vi "CRYCalcu Arithmetic Value.vi"(4 "dB ref":dbl format="%#_6p", 5 "Axis Mode":u16(slide), 6 "B data for units":T1={"Name"="", "Curve"=[], "X data"=1, "Y data"=1, "Z data"=1, "X axis"=0, "Y axis"=1, "Z axis"=1, "X unit"="Hz", "Y unit"="", "Z unit"="deg.", "X dB ref"=1.0, "Y dB ref"=1.0, "Z dB ref"=1.0, "single val"=FALSE, "protected"=FALSE, "display X"=TRUE, "display Y"=TRUE, "display Z"=TRUE, "Test Info"="", "Step No."=0, "Plot Settings"={"Color"=0, "Interpolation"=0, "Point Style"=0, "Line Style"=0, "Point Color"=0, "Line Width"=0, "Bar Plot Style"=0, "Fill To"=0}, "AutoProtect"=FALSE} {"Z data" items=["dB", "Lin"]; "X data" items=["dB", "Lin"]; "Y data" items=["dB", "Lin"]; "Z dB ref" format="%.1f"; "Z axis" items=["Log", "Lin"]; "X dB ref" format="%.1f"; "X axis" items=["Log", "Lin"]; "Y axis" items=["Log", "Lin"]; "Y dB ref" format="%.1f"; "Curve"."z" format="%.2f"; "Curve"."y" format="%.2f"; "Curve"."x" format="%.2f"}, 7 "A data for units":T1={"Name"="", "Curve"=[], "X data"=1, "Y data"=1, "Z data"=1, "X axis"=0, "Y axis"=1, "Z axis"=1, "X unit"="Hz", "Y unit"="", "Z unit"="deg.", "X dB ref"=1.0, "Y dB ref"=1.0, "Z dB ref"=1.0, "single val"=FALSE, "protected"=FALSE, "display X"=TRUE, "display Y"=TRUE, "display Z"=TRUE, "Test Info"="", "Step No."=0, "Plot Settings"={"Color"=0, "Interpolation"=0, "Point Style"=0, "Line Style"=0, "Point Color"=0, "Line Width"=0, "Bar Plot Style"=0, "Fill To"=0}, "AutoProtect"=FALSE} {"Z data" items=["dB", "Lin"]; "X data" items=["dB", "Lin"]; "Y data" items=["dB", "Lin"]; "Z dB ref" format="%.1f"; "Z axis" items=["Log", "Lin"]; "X dB ref" format="%.1f"; "X axis" items=["Log", "Lin"]; "Y axis" items=["Log", "Lin"]; "Y dB ref" format="%.1f"; "Curve"."z" format="%.2f"; "Curve"."y" format="%.2f"; "Curve"."x" format="%.2f"}, 8 "Curve B":cluster{"x":dbl, "y":dbl, "z":dbl}[](array[cluster]) {"z" format="%.2f"; "y" format="%.2f"; "x" format="%.2f"}, 9 "operator":u16(ring) items=["+", "--", "x", "/"], 10 "Work in":u16(slide), 11 "Curve A":cluster{"x":dbl, "y":dbl, "z":dbl}[](array[cluster]) {"z" format="%.2f"; "y" format="%.2f"; "x" format="%.2f"}) -> (2 "Result":cluster{"x":dbl, "y":dbl, "z":dbl}[](array[cluster]) {"z" format="%.2f"; "y" format="%.2f"; "x" format="%.2f"})   [LabVIEW 2013]
uses:
  Typedef Control/CRYData Cluster.ctl
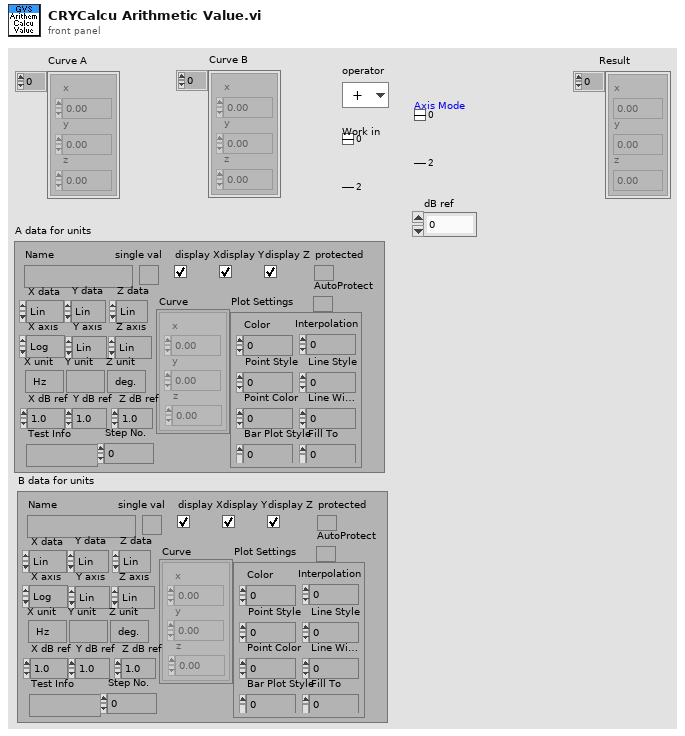
[diagram p1: front panel]
types:
  T1 = typedef "CRYData Cluster.ctl" = cluster{"Name":string, "Curve":cluster{"x":dbl, "y":dbl, "z":dbl}[], "X data":u16, "Y data":u16, "Z data":u16, "X axis":u16, "Y axis":u16, "Z axis":u16, "X unit":string, "Y unit":string, "Z unit":string, "X dB ref":dbl, "Y dB ref":dbl, "Z dB ref":dbl, "single val":bool, "protected":bool, "display X":bool, "display Y":bool, "display Z":bool, "Test Info":string, "Step No.":i32, "Plot Settings":cluster{"Color":u32, "Interpolation":u8, "Point Style":u8, "Line Style":u8, "Point Color":u32, "Line Width":u8, "Bar Plot Style":u8, "Fill To":i16}, "AutoProtect":bool}
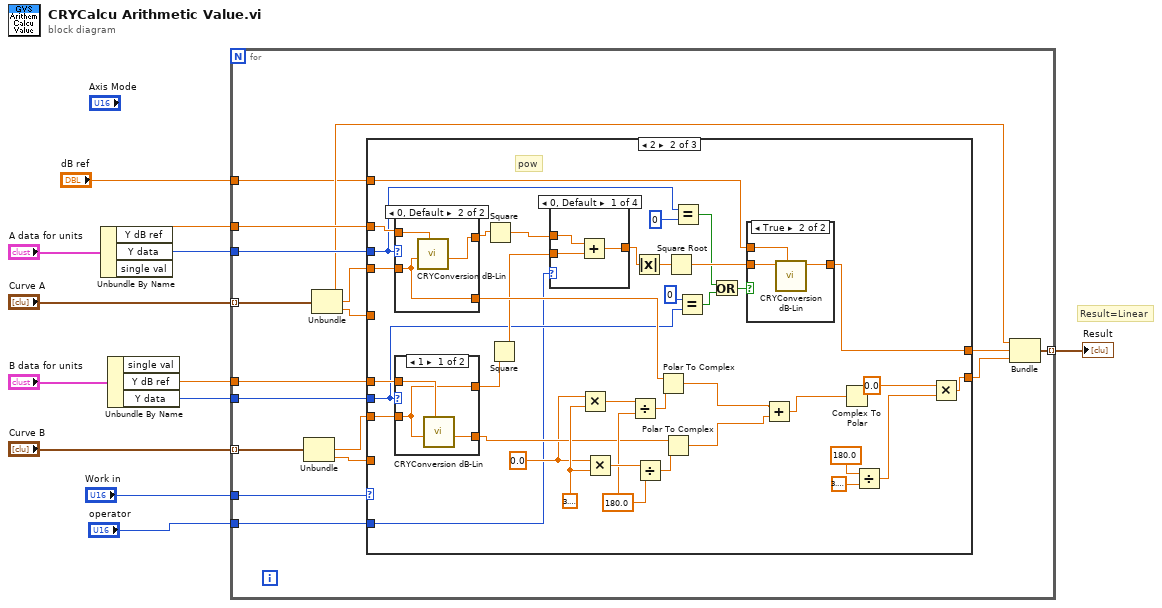
[diagram p0: block diagram]
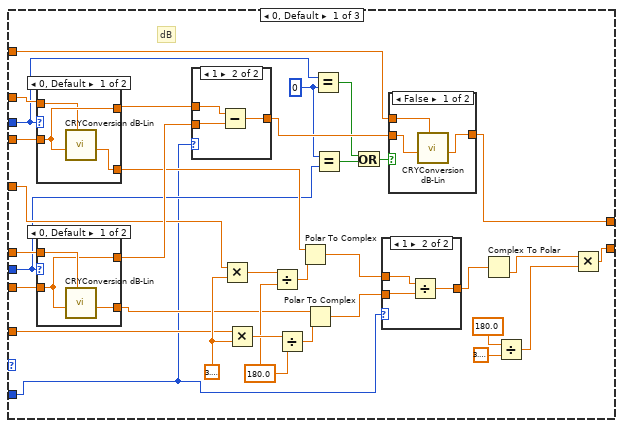
[diagram p2: hidden frame]
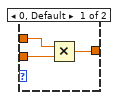
[diagram p4: hidden frame]
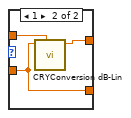
[diagram p5: hidden frame]
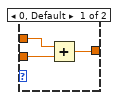
[diagram p6: hidden frame]
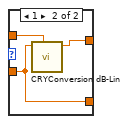
[diagram p7: hidden frame]
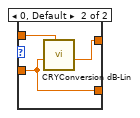
[diagram p9: hidden frame]
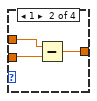
[diagram p10: hidden frame]
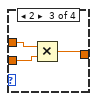
[diagram p11: hidden frame]
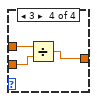
[diagram p12: hidden frame]
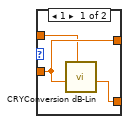
[diagram p13: hidden frame]
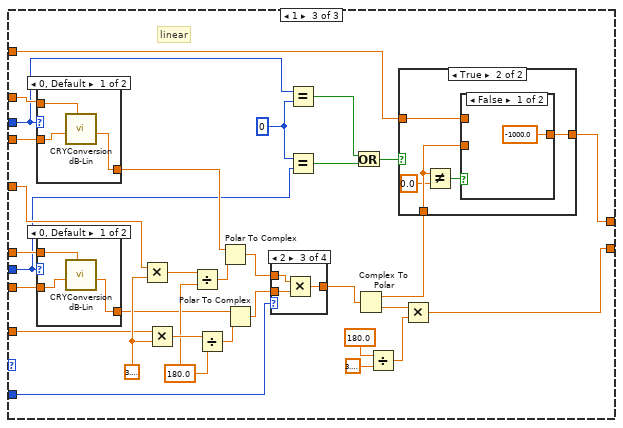
[diagram p14: hidden frame]
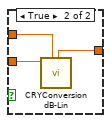
[diagram p16: hidden frame]
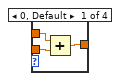
[diagram p17: hidden frame]
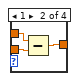
[diagram p18: hidden frame]
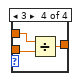
[diagram p19: hidden frame]
diagram:
  # "Result=Linear"
  n1 = Unbundle By Name("A data for units") -> ("Y dB ref"=w6:dbl, "Y data"=w7:u16)  [unwired: 1 out]
  n2 = Unbundle By Name("B data for units") -> ("Y dB ref"=w4:dbl, "Y data"=w5:u16)  [unwired: 1 out]
  n3 = for {
    tunnel: "Curve B" -> [w29] mode=indexing
    tunnel: "Curve A" -> [w28] mode=indexing
    tunnel: [w27] -> w11 mode=indexing
    tunnel: w7 -> [w26]
    tunnel: w6 -> [w25]
    tunnel: w5 -> [w24]
    tunnel: w4 -> [w23]
    tunnel: "dB ref" -> [w16]
    tunnel: "Work in" -> [w14]
    tunnel: "operator" -> [w13]
    n4 = Unbundle(w29) -> ("y"=w21:dbl, "z"=w18:dbl)  [unwired: 1 out]
    n5 = Unbundle(w28) -> ("x"=w17:dbl, "y"=w22:dbl, "z"=w19:dbl)
    n6 = case shown="2" w14 {
      tunnel: w22 -> [w56 w122 w184]
      tunnel: w21 -> [w59 w125 w185]
      tunnel: w13 -> [w30 w92 w158]
      tunnel: w26 -> [w35 w99 w163]
      tunnel: w25 -> [w61 w127 w187]
      tunnel: w24 -> [w34 w97 w162]
      tunnel: w23 -> [w60 w126 w186]
      tunnel: [w43 w113 w172] -> w20
      tunnel: w19 -> [w49 _ w177]
      tunnel: w18 -> [w48 _ w176]
      tunnel: [w38 w109 w165] -> w15
      tunnel: w16 -> [w42 w112 w171]
      frame 0, Default {
        w33 = u16 0 ("y")
        w52 = 180.0
        w53 = 3.141592653589793
        # "dB"
        n7 = case shown="0, Default" w35 {
          tunnel: [w88 w90] -> w58
          tunnel: w56 -> [w88 w89]
          tunnel: w61 -> [w87 w91]
          tunnel: [w86 w89] -> w50
          frame 0, Default {
            n8 = call "CRYConversion dB-Lin.vi"("dB ref."=w87, "Log In"=w88) -> ("Lin Out"=w86:dbl)  [unwired: 4 in, 3 out]
          }
          frame 1 {
            n9 = call "CRYConversion dB-Lin.vi"("dB ref."=w91, "Lin In"=w89) -> ("Log Out"=w90:dbl)  [unwired: 4 in, 3 out]
          }
        }
        n10 = case shown="0, Default" w34 {
          tunnel: [w75 w78] -> w57
          tunnel: w59 -> [w75 w77]
          tunnel: w60 -> [w76 w79]
          tunnel: [w74 w77] -> w51
          frame 0, Default {
            n11 = call "CRYConversion dB-Lin.vi"("dB ref."=w76, "Log In"=w75) -> ("Lin Out"=w74:dbl)  [unwired: 4 in, 3 out]
          }
          frame 1 {
            n12 = call "CRYConversion dB-Lin.vi"("dB ref."=w79, "Lin In"=w77) -> ("Log Out"=w78:dbl)  [unwired: 4 in, 3 out]
          }
        }
        n13 = case shown="1" w30 {
          tunnel: [w82 w85] -> w44
          tunnel: w58 -> [w81 w84]
          tunnel: w57 -> [w80 w83]
          frame 0, Default {
            n14 = Add(x=w81, y=w80) -> (x+y=w82:dbl)
          }
          frame 1 {
            n15 = Subtract(x=w84, y=w83) -> (x-y=w85:dbl)
          }
        }
        n16 = Multiply(x=w49, y=w53) -> (x*y=w55:dbl)
        n17 = Multiply(x=w48, y=w53) -> (x*y=w62:dbl)
        n18 = Divide(x=w55, y=w52) -> (x/y=w54:dbl)
        n19 = Divide(x=w62, y=w52) -> (x/y=w63:dbl)
        n20 = Polar To Complex(1:w54, 2:w50) -> (0:w47:cdb)
        n21 = Polar To Complex(1:w63, 2:w51) -> (0:w46:cdb)
        n22 = Equal?(x=w35, y=w33) -> (x = y?=w31:bool)
        n23 = Equal?(x=w33, y=w34) -> (x = y?=w32:bool)
        n24 = Or(x=w31, y=w32) -> (x .or. y?=w45:bool)
        n25 = case shown="1" w30 {
          tunnel: [w70 w73] -> w39
          tunnel: w47 -> [w69 w72]
          tunnel: w46 -> [w68 w71]
          frame 0, Default {
            n26 = Multiply(x=w69, y=w68) -> (x*y=w70:cdb)
          }
          frame 1 {
            n27 = Divide(x=w72, y=w71) -> (x/y=w73:cdb)
          }
        }
        n28 = case shown="False" w45 {
          tunnel: [w64 w67] -> w43
          tunnel: w44 -> [w65 w67]
          tunnel: w42 -> [w66 _]
          frame False {
            n29 = call "CRYConversion dB-Lin.vi"("dB ref."=w66, "Log In"=w65) -> ("Lin Out"=w64:dbl)  [unwired: 4 in, 3 out]
          }
          frame True {
          }
        }
        n30 = Complex To Polar(r * e^(i*theta)=w39) -> (theta=w37:dbl)  [unwired: 1 out]
        n31 = Divide(x=180.0, y=3.141592653589793) -> (x/y=w36:dbl)
        n32 = Multiply(x=w37, y=w36) -> (x*y=w38:dbl)
      }
      frame 2 {
        w104 = 0.0 ("x")
        w118 = 180.0
        w119 = 3.141592653589793
        # "pow"
        n33 = case shown="0, Default" w99 {
          tunnel: [w154 w155] -> w124
          tunnel: w122 -> [w154 w156]
          tunnel: w127 -> [w153 w157]
          tunnel: [w152 w156] -> w116
          frame 1 {
            n34 = call "CRYConversion dB-Lin.vi"("dB ref."=w153, "Log In"=w154) -> ("Lin Out"=w152:dbl)  [unwired: 4 in, 3 out]
          }
          frame 0, Default {
            n35 = call "CRYConversion dB-Lin.vi"("dB ref."=w157, "Log In"=w156) -> ("Lin Out"=w155:dbl)  [unwired: 4 in, 3 out]
          }
        }
        n36 = case shown="1" w97 {
          tunnel: [w135 w137] -> w123
          tunnel: w125 -> [w135 w138]
          tunnel: w126 -> [w136 w139]
          tunnel: [w134 w138] -> w117
          frame 1 {
            n37 = call "CRYConversion dB-Lin.vi"("dB ref."=w136, "Log In"=w135) -> ("Lin Out"=w134:dbl)  [unwired: 4 in, 3 out]
          }
          frame 0, Default {
            n38 = call "CRYConversion dB-Lin.vi"("dB ref."=w139, "Log In"=w138) -> ("Lin Out"=w137:dbl)  [unwired: 4 in, 3 out]
          }
        }
        n39 = Square(x=w124) -> (x^2=w103:dbl)
        n40 = Square(x=w123) -> (x^2=w102:dbl)
        n41 = case shown="0, Default" w92 {
          tunnel: [w142 w145 w146 w149] -> w114
          tunnel: w103 -> [w141 w144 w148 w151]
          tunnel: w102 -> [w140 w143 w147 w150]
          frame 0, Default {
            n42 = Add(x=w141, y=w140) -> (x+y=w142:dbl)
          }
          frame 1 {
            n43 = Subtract(x=w144, y=w143) -> (x-y=w145:dbl)
          }
          frame 2 {
            n44 = Multiply(x=w148, y=w147) -> (x*y=w146:dbl)
          }
          frame 3 {
            n45 = Divide(x=w151, y=w150) -> (x/y=w149:dbl)
          }
        }
        n46 = Multiply(x=w104, y=w119) -> (x*y=w121:dbl)
        n47 = Multiply(x=w104, y=w119) -> (x*y=w128:dbl)
        n48 = Divide(x=w121, y=w118) -> (x/y=w120:dbl)
        n49 = Absolute Value(x=w114) -> (abs(x)=w101:dbl)
        n50 = Divide(x=w128, y=w118) -> (x/y=w129:dbl)
        n51 = Polar To Complex(1:w120, 2:w116) -> (0:w107:cdb)
        n52 = Polar To Complex(1:w129, 2:w117) -> (0:w106:cdb)
        n53 = Square Root(x=w101) -> (sqrt(x)=w100:dbl)
        n54 = Equal?(x=w99, y=u16 0) -> (x = y?=w94:bool)
        n55 = Equal?(x=u16 0, y=w97) -> (x = y?=w95:bool)
        n56 = Or(x=w94, y=w95) -> (x .or. y?=w115:bool)
        n57 = case shown="True" w115 {
          tunnel: [w130 w131] -> w113
          tunnel: w100 -> [w130 w133]
          tunnel: w112 -> [_ w132]
          frame False {
          }
          frame True {
            n58 = call "CRYConversion dB-Lin.vi"("dB ref."=w132, "Lin In"=w133) -> ("Log Out"=w131:dbl)  [unwired: 4 in, 3 out]
          }
        }
        n59 = Add(x=w107, y=w106) -> (x+y=w105:cdb)
        n60 = Complex To Polar(r * e^(i*theta)=w105) -> ()  [unwired: 2 out]
        n61 = Divide(x=180.0, y=3.141592653589793) -> (x/y=w108:dbl)
        n62 = Multiply(x=0.0, y=w108) -> (x*y=w109:dbl)
      }
      frame 1 {
        w161 = u16 0 ("x")
        w180 = 180.0
        w181 = 3.141592653589793
        # "linear"
        n63 = case shown="0, Default" w163 {
          tunnel: w184 -> [w218 w219]
          tunnel: w187 -> [w217 _]
          tunnel: [w216 w219] -> w178
          frame 0, Default {
            n64 = call "CRYConversion dB-Lin.vi"("dB ref."=w217, "Log In"=w218) -> ("Lin Out"=w216:dbl)  [unwired: 4 in, 3 out]
          }
          frame 1 {
          }
        }
        n65 = case shown="0, Default" w162 {
          tunnel: w185 -> [w213 w215]
          tunnel: w186 -> [w214 _]
          tunnel: [w212 w215] -> w179
          frame 0, Default {
            n66 = call "CRYConversion dB-Lin.vi"("dB ref."=w214, "Log In"=w213) -> ("Lin Out"=w212:dbl)  [unwired: 4 in, 3 out]
          }
          frame 1 {
          }
        }
        n67 = Multiply(x=w177, y=w181) -> (x*y=w183:dbl)
        n68 = Multiply(x=w176, y=w181) -> (x*y=w188:dbl)
        n69 = Divide(x=w183, y=w180) -> (x/y=w182:dbl)
        n70 = Divide(x=w188, y=w180) -> (x/y=w189:dbl)
        n71 = Polar To Complex(1:w182, 2:w178) -> (0:w175:cdb)
        n72 = Polar To Complex(1:w189, 2:w179) -> (0:w174:cdb)
        n73 = case shown="2" w158 {
          tunnel: [w202 w205 w206 w211] -> w166
          tunnel: w175 -> [w201 w204 w208 w210]
          tunnel: w174 -> [w200 w203 w207 w209]
          frame 0, Default {
            n74 = Add(x=w201, y=w200) -> (x+y=w202:cdb)
          }
          frame 1 {
            n75 = Subtract(x=w204, y=w203) -> (x-y=w205:cdb)
          }
          frame 2 {
            n76 = Multiply(x=w208, y=w207) -> (x*y=w206:cdb)
          }
          frame 3 {
            n77 = Divide(x=w210, y=w209) -> (x/y=w211:cdb)
          }
        }
        n78 = Equal?(x=w163, y=w161) -> (x = y?=w160:bool)
        n79 = Equal?(x=w161, y=w162) -> (x = y?=w159:bool)
        n80 = Or(x=w160, y=w159) -> (x .or. y?=w173:bool)
        n81 = Complex To Polar(r * e^(i*theta)=w166) -> (r=w164:dbl, theta=w168:dbl)
        n82 = Divide(x=180.0, y=3.141592653589793) -> (x/y=w167:dbl)
        n83 = case shown="True" w173 {
          tunnel: [w190 w194] -> w172
          tunnel: w171 -> [_ w195]
          tunnel: w164 -> [w190 w193]
          frame False {
          }
          frame True {
            n84 = Not Equal?(x=w193, y=0.0) -> (x != y?=w191:bool)
            n85 = case shown="False" w191 {
              tunnel: w195 -> [_ w199]
              tunnel: [-1000.0 ("Log Out") w198] -> w194
              tunnel: w193 -> [_ w197]
              frame False {
              }
              frame True {
                n86 = call "CRYConversion dB-Lin.vi"("dB ref."=w199, "Lin In"=w197) -> ("Log Out"=w198:dbl)  [unwired: 4 in, 3 out]
              }
            }
          }
        }
        n87 = Multiply(x=w168, y=w167) -> (x*y=w165:dbl)
      }
    }
    n88 = Bundle("x"=w17, "Log Out"=w20, w15) -> (w27:cluster{"x":dbl, "Log Out":dbl, dbl})  [unwired: 1 in]
  }
  "Result" <- w11
